vi "OCT Reference Follower.vi"(6 "stop":bool, 7 "OCT Act ON":bool=TRUE, 8 "OCT Z PID Gains":cluster{"Kp":dbl, "Kd":dbl, "Ki":dbl}={"Kp"=0.0003, "Kd"=0.0001, "Ki"=0.01}, 9 "OCT  Z cmd Posit [mm]":dbl, 10 "error in":errorcluster, 11 "FPGA VI Reference In":refnum<k20>) -> (1 "OCT  Z out Posit [mm]":dbl, 2 "error out":errorcluster, 3 "FPGA VI Reference Out":refnum<k20>)   [LabVIEW 2016]
uses:
  <vilib>/rvi/errors/niLvFpgaAdjustHostInterfaceError.vi
  <vilib>/Utility/error.llb/Error Cluster From Error Code.vi
  <vilib>/rvi/interface/nirviReadWriteControl/nirviReadWriteControl.xnode
  FPGA Bitfiles/PhantomControlPI_FPGATarget_QuadCtr2_E2412E44.lvbitx
  IRISS_FPGA_IO.vi
  Library/jmslib.lvlib
  <vilib>/rvi/interface/nirviOpenFPGA/nirviOpenFPGA.xnode
  <vilib>/FPGAPlugInAG/PXI-7833R/niLvFpga_Open_PXI-7833R.vi
  NiFpgaLv.dll
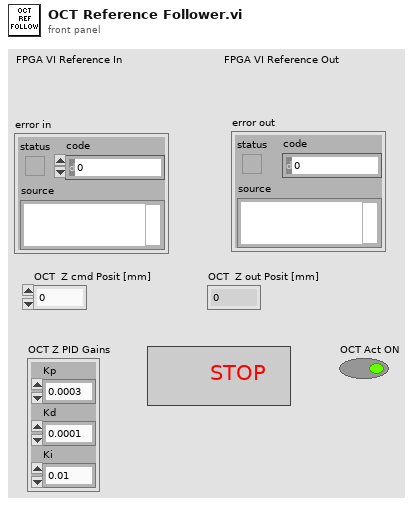
[diagram p1: front panel]
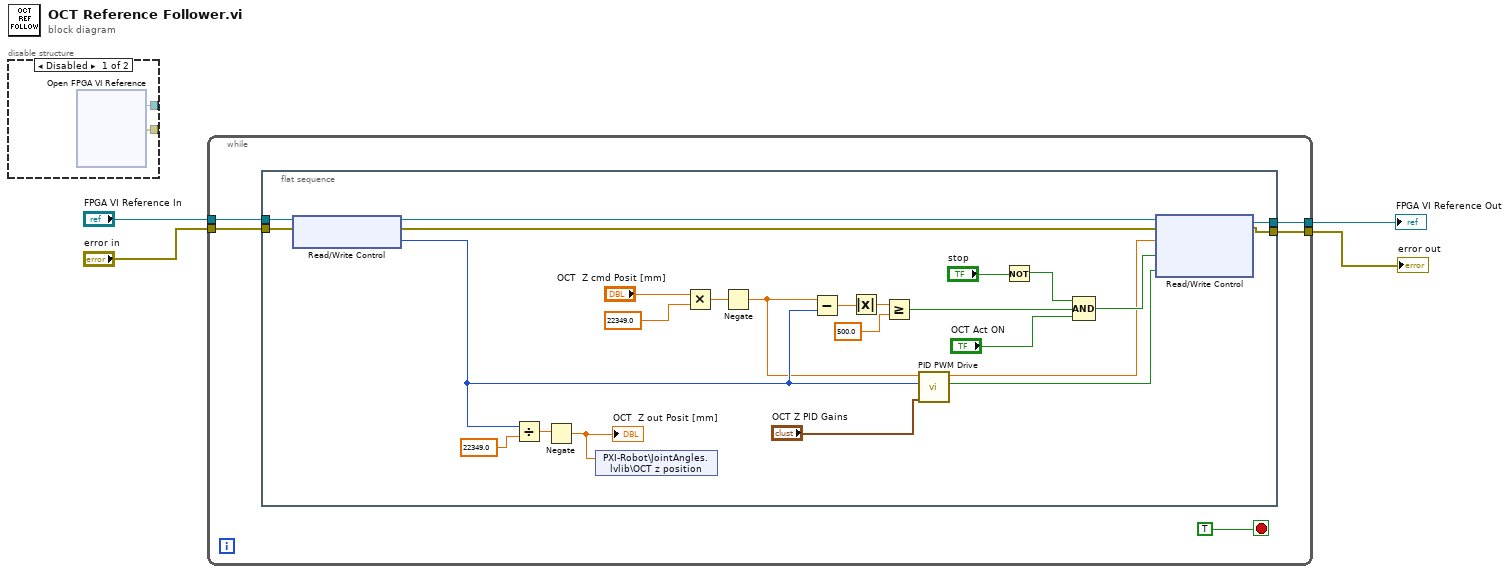
[diagram p0: block diagram]
diagram:
  n1 = disable-structure shown="Disabled" {
    disable-tunnel: [w6 _] -> _
    disable-tunnel: [w5 _] -> _
    frame Disabled {
      n2 = xnode "Open FPGA VI Reference"() -> ("FPGA VI Reference Out"=w6:refnum<k20>, "error out"=w5:errorcluster)  [unwired: 2 in]
    }
    frame Enabled {
    }
  }
  n3 = while {
    tunnel: "FPGA VI Reference In" -> [w11]
    tunnel: "error in" -> [w10]
    tunnel: [w9] -> w3
    tunnel: [w8] -> w4
    stop <- TRUE ("Boolean") stop-if-true
    n4 = flat-sequence {
      tunnel: w11 -> [w36]
      tunnel: w10 -> [w35]
      tunnel: [w34] -> w9
      tunnel: [w33] -> w8
      frame #0 {
        n5 = xnode "Read/Write Control"("FPGA VI Reference In"=w36, "error in"=w35) -> ("FPGA VI Reference Out"=w31:refnum<k20>, "error out"=w30:errorcluster, "32 bit Position 14"=w16:i32)
        n6 = Divide(x=w16, y=22349.0) -> (x/y=w15:dbl)
        n7 = Negate(x=w15) -> (-x=w14:dbl)
        "OCT  Z out Posit [mm]" <- w14
        n8 = shared-variable "PXI-Robot\\JointAngles.lvlib\\OCT z position"(w14) -> ()  [unwired: 1 in, 1 out]
        n9 = Multiply(x="OCT  Z cmd Posit [mm]", y=22349.0) -> (x*y=w13:dbl)
        n10 = Negate(x=w13) -> (-x=w12:dbl)
        n11 = Subtract(x=w12, y=w16) -> (x-y=w29:dbl)
        n12 = Absolute Value(x=w29) -> (abs(x)=w28:dbl)
        n13 = Greater Or Equal?(x=w28, y=500.0) -> (x >= y?=w22:bool)
        n14 = call "PID PWM Drive.vi"("PID Gains"="OCT Z PID Gains", "Encoder Position"=w16, "Reference"=w12) -> ("Direction"=w21:bool, "Duty Cycle"=w19:dbl)  [unwired: 6 in, 1 out]
        n15 = Not(x="stop") -> (.not. x?=w32:bool)
        n16 = Compound Arithmetic op=AND(w32, w22, "OCT Act ON") -> (w20:bool)
        n17 = xnode "Read/Write Control"("FPGA VI Reference In"=w31, "error in"=w30, "OCT Mot DC"=w19, "INHB OCT Mot"=w20, "DIR OCT Mot"=w21) -> ("FPGA VI Reference Out"=w34:refnum<k20>, "error out"=w33:errorcluster)
      }
    }
  }
  "error out" <- w4
  "FPGA VI Reference Out" <- w3
